vi "Trial Config Parameter Guide.vi"(8 "Error IN":errorcluster) -> (0 "Error OUT":errorcluster)   [LabVIEW 2018]
panel:
  in  "Close":bool
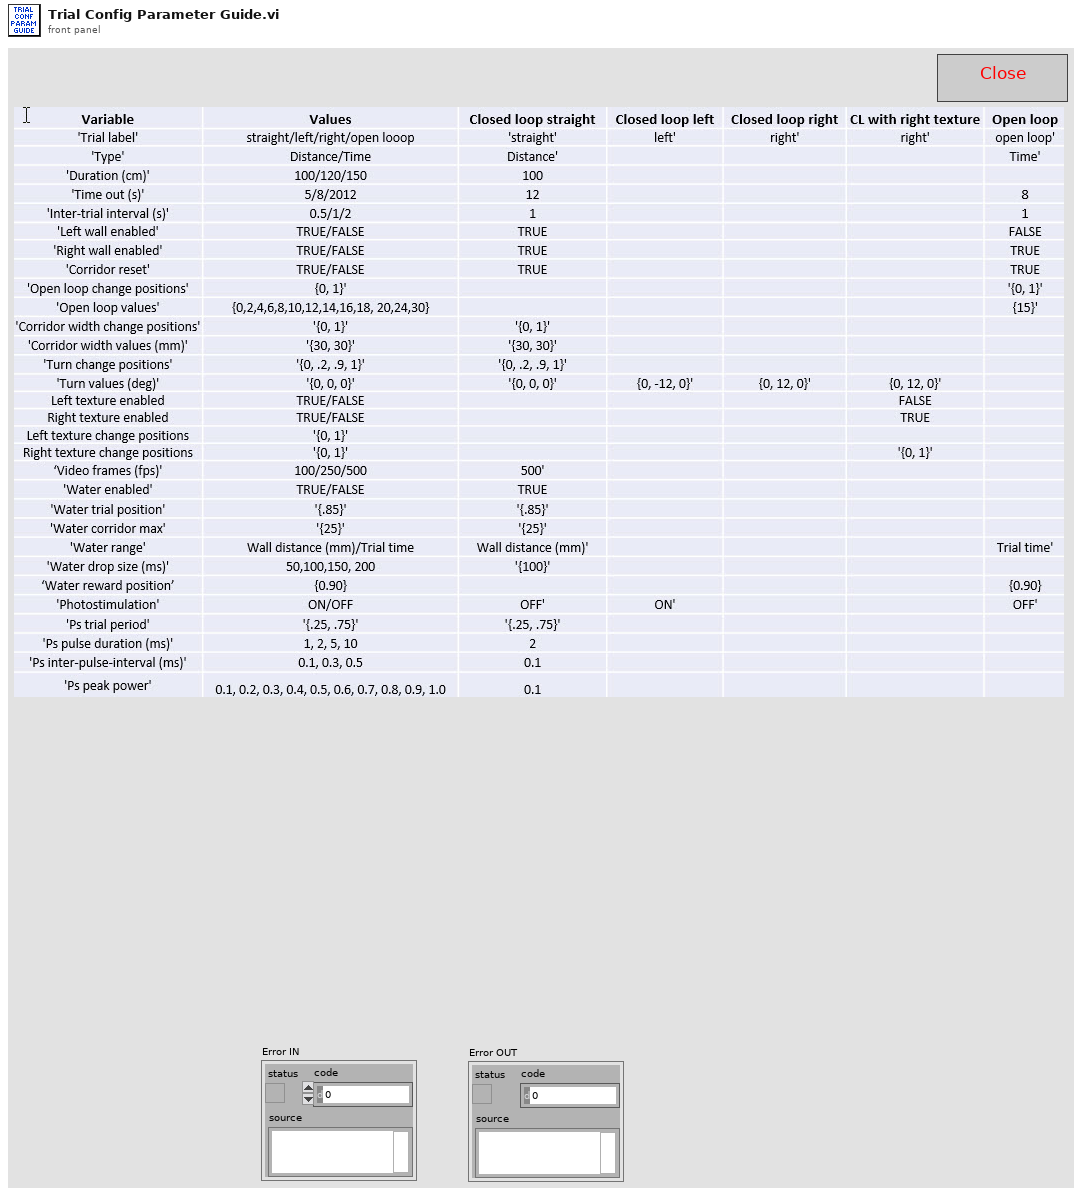
[diagram p1: front panel]
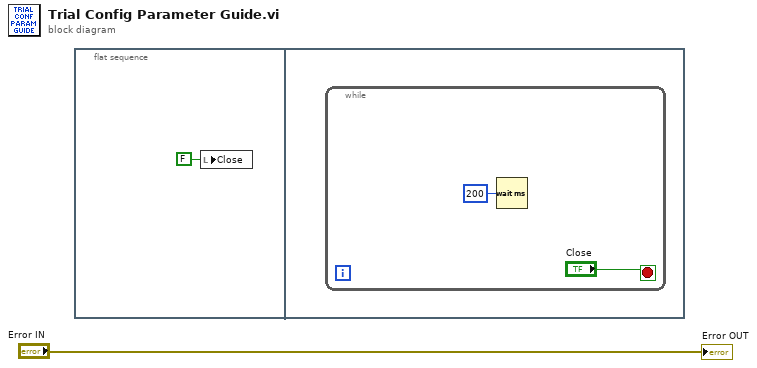
[diagram p0: block diagram]
diagram:
  n1 = flat-sequence {
    frame #0 {
      n2 = local write "Close"(FALSE ("Close")) -> ()
    }
    frame #1 {
      n3 = while {
        stop <- "Close" stop-if-true
        n4 = Wait (ms)(milliseconds to wait=u32 200) -> ()  [unwired: 1 out]
      }
    }
  }
  "Error OUT" <- "Error IN"
